vi "Fibonacci_Series.vi"() -> ()   [LabVIEW 2024]
panel:
  in  "Numeric":i32
  out "Array":i32[](array[numeric])
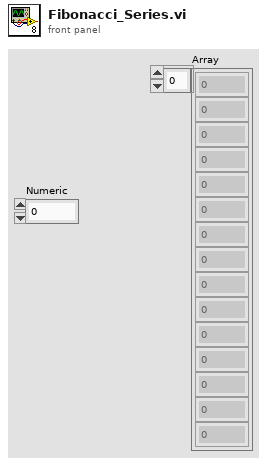
[diagram p1: front panel]
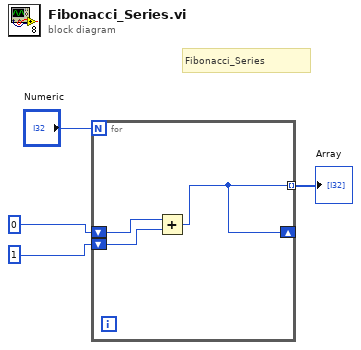
[diagram p0: block diagram]
diagram:
  # "Fibonacci_Series"
  n1 = for {
    N: "Numeric" -> [_]
    shift-right: [w5] -> _
    shift-left: 1 -> [w7]
    shift-left: 0 -> [w6]
    tunnel: [w5] -> w2 mode=indexing
    n2 = Add(x=w6, y=w7) -> (x+y=w5:i32)
  }
  "Array" <- w2
